vi "GetMatlabBoundControlCollection.vi"(11 "ExpID":string) -> (3 "Bound Controls":T1[](array[typedef]))   [LabVIEW 2017]
uses:
  Types/ControlValueChangeEventBindingType.ctl
  Types/MatlabBindingDirectionEnum.ctl
  MatlabGlobals.vi
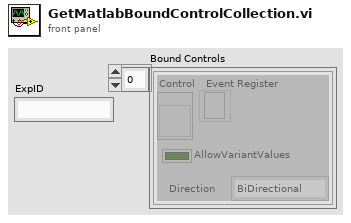
[diagram p1: front panel]
types:
  T1 = typedef "ControlValueChangeEventBindingType.ctl" = cluster{"Control":refnum<vi>, "Event Register":refnum<event-registration>, "AllowVariantValues":bool, "Direction":T2}
  T2 = typedef "MatlabBindingDirectionEnum.ctl" = enum16{"BiDirectional", "FromMatlab", "ToMatlab"}
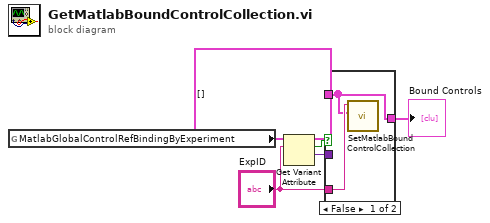
[diagram p0: block diagram]
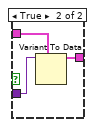
[diagram p2: hidden frame]
diagram:
  n1 = global read "MatlabGlobals.vi" "MatlabGlobalControlRefBindingByExperiment"() -> (w4:variant)
  n2 = Get Variant Attribute(Variant=w4, name="ExpID") -> (found=w2:bool, value=w6:variant)  [unwired: 2 in, 2 out]
  n3 = case shown="False" w2 {
    tunnel: w6 -> [_ w11]
    tunnel: T1[] [] -> [w7 w10]
    tunnel: [w7 w9] -> w3
    tunnel: "ExpID" -> [w8 _]
    frame False {
      n4 = call "SetMatlabBoundControlCollection.vi"("Bound controls"=w7, "ExpID"=w8) -> ()  [unwired: 10 in]
    }
    frame True {
      n5 = Variant To Data(type=w10, Variant=w11) -> (data=w9:T1[])  [unwired: 1 in, 1 out]
    }
  }
  "Bound Controls" <- w3
